vi "FailureDescription.vi"(8 "error in (no error)":errorcluster, 10 "Actual":variant, 11 "IsType in":refnum<class "IsType.lvclass">) -> (0 "error out":errorcluster, 2 "Failure Description":string, 3 "IsType out":refnum<class "IsType.lvclass">)   [LabVIEW 2017, in "Constraint.lvlib" / "IsType.lvclass"]
doc: "Return the second part of the scentence \"Failed asserting that ...\""
uses:
  IsType.lvclass
  <vilib>/Utility/Data Type/NI_Data Type.lvlib
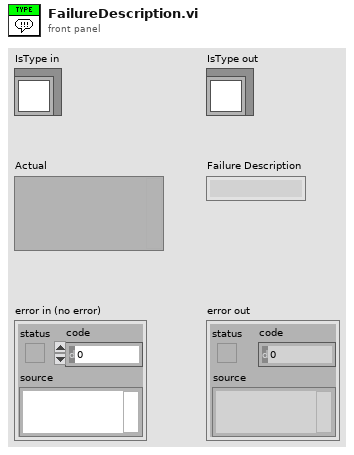
[diagram p1: front panel]
types:
  T1 = typedef "NI_Data Type.lvlib/Data Type.ctl" = enum8{"Invalid Type", "Void", "I8", "I16", "I32", "I64", "U8", "U16", "U32", "U64", "Single Float", "Double Float", "Extended Float", "Single Complex", "Double Complex", "Extended Complex", "Enum U8", "Enum U16", "Enum U32", "Enum U64", "Single Float With Unit", "Double Float With Unit", "Extended Float With Unit", "Single Complex with Unit", "Double Complex with Unit", "Extended Complex with Unit", "Boolean", "String", "Path", "Picture", "Tag", "Array", "Cluster", "Variant", "LV Variant", "Waveform", "Timestamp", "Digital Waveform", "Digital Data", "ExpressData", "Refnum", "External Data", "VI", "Poly VI", "LabVIEW Class Instance", "Fixed Point", "Set Collection", "Map Collection"}
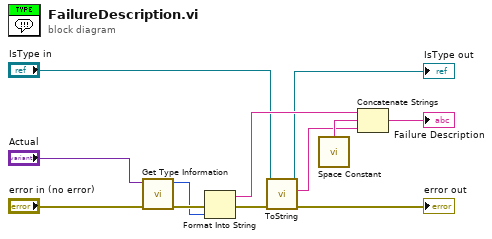
[diagram p0: block diagram]
diagram:
  n1 = call <vilib>:"Get Type Information.vi"("error in (no error)"="error in (no error)", "variant"="Actual") -> ("error out"=w9:errorcluster, "type"=w6:T1)  [unwired: 5 in, 3 out]
  n2 = Format Into String(error in=w9, w6) -> (resulting string=w5:string, error out=w7:errorcluster)  [unwired: 2 in]
  n3 = call-dynamic "ToString.vi"("error in (no error)"=w7, "IsType in"="IsType in") -> ("error out"=→"error out":errorcluster, "String"=w11:string, "IsType out"=→"IsType out":refnum<class "IsType.lvclass">)  [unwired: 7 in]
  n4 = call <vilib>:"Space Constant.vi"() -> ("String"=w12:string)
  n5 = Concatenate Strings(w5, w12, w11) -> (→"Failure Description":string)
